vi "Microscopy.Circular Buffer (BRAM)_Array_Multi-Channel.vi"(0 "Input Write Data":T2=[0, 0, 0, 0], 1 "Acquisition Status In":T1, 2 "Read Data?":bool, 3 "Input Valid":bool, 5 "Acq Param Pre Trigger Samples":u16) -> (7 "Output Write Data":T2, 9 "Acquisition Status Out":T1, 10 "Output Valid":bool)   [LabVIEW 2014]
doc: "This VI maintains a circular buffer with user configurable buffer size.\nMaximum Buffer Size = 4096 (U32) elements\n\n<b> Delay = 1 Tick </b>"
uses:
  Adapter Module Specific/Multi-Channel Analog Input Data.ctl
  Acquisition Status.ctl
  <vilib>/Utility/error.llb/Clear Errors.vi
  <vilib>/rvi/Emulation/niFpgaSctlEmulationGetInTimedLoop.vi
  <vilib>/rvi/DataTransferAndStorage/Container/Common/niFpgaContainerGetUniqueNameForEmu.vi
  <vilib>/rvi/DataTransferAndStorage/Container/Common/niFpgaContainerSetEmuInfo.vi
  <vilib>/rvi/eio/common/nirviEmuReportErrorAndStop.vi
  <vilib>/rvi/Memory/Memory_Emulation/nirvimemoryEmulation.vi
  <vilib>/rvi/Memory/Memory_Emulation/nirvimemoryFastEmulation.vi
  <vilib>/rvi/Memory/Memory_Emulation/niFpgaMemoryEmulationCacheClearOnFirstRun.vi
  <vilib>/rvi/Memory/Memory_Emulation/nirvimemoryEmulationManagerCache_MakeExclusive.vi
  <vilib>/rvi/Memory/Memory_Emulation/niFpgaMemoryEmulationValidateCache.vi
  <vilib>/rvi/Memory/Memory_Emulation/nirvimemoryEmulationManagerCache_InsertValue.vi
  <vilib>/rvi/Memory/Memory_Emulation/nirvimemoryEmulationManagerCache_ReleaseExclusive.vi
  <vilib>/rvi/Memory/Memory_Emulation/nirvimemoryEmulationManagerCache_GetValue.vi
  <vilib>/rvi/Emulation/niFpgaEmulationIsFPGAContextNoSignature.vi
  <vilib>/rvi/Memory/Memory_Emulation/nirvimemoryEmulationManagerCache_SetValue.vi
  <vilib>/rvi/Emulation/niFpgaSctlEmulationResourceMgr.vi
  <vilib>/rvi/LocalResourceManager/LocalResourceManager.xnode
  <vilib>/rvi/DataTransferAndStorage/Container/XNode/niFpgaContainer.xnode
panel:
  # "Copyright 2014 Vidrio Technologies\nScanImage 5 software is licensed under the Apache License, Version 2.0 (the \"License\"); you may not use any files contained\nwithin the ScanImage 5 release except in compliance with the License. You may obtain a copy of the License at\n http://www.apache.org/licenses/LICENSE-2.0\nUnless required by applicable law or agreed to in writing, software distributed under the License is distributed on an\n\"AS IS\" BASIS, WITHOUT WARRANTIES OR CONDITIONS OF ANY KIND, either express or implied. See the License for the\n specific language governing permissions and limitations under the License."
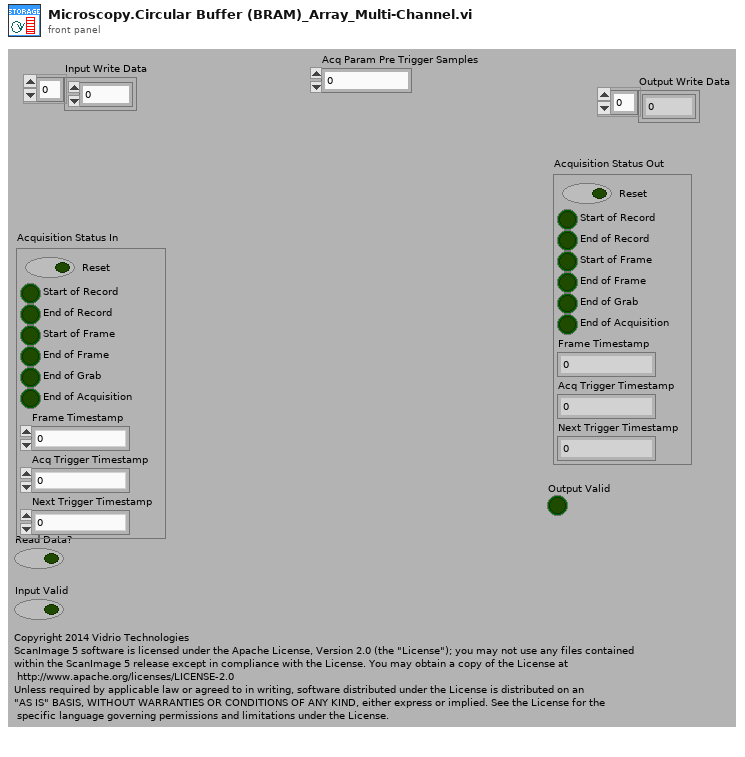
[diagram p1: front panel]
types:
  T1 = typedef "Acquisition Status.ctl" = cluster{"Reset":bool, "Start of Record":bool, "End of Record":bool, "Start of Frame":bool, "End of Frame":bool, "End of Grab":bool, "End of Acquisition":bool, "Frame Timestamp":u64, "Acq Trigger Timestamp":u64, "Next Trigger Timestamp":u64}
  T2 = typedef "Multi-Channel Analog Input Data.ctl" = i16[]
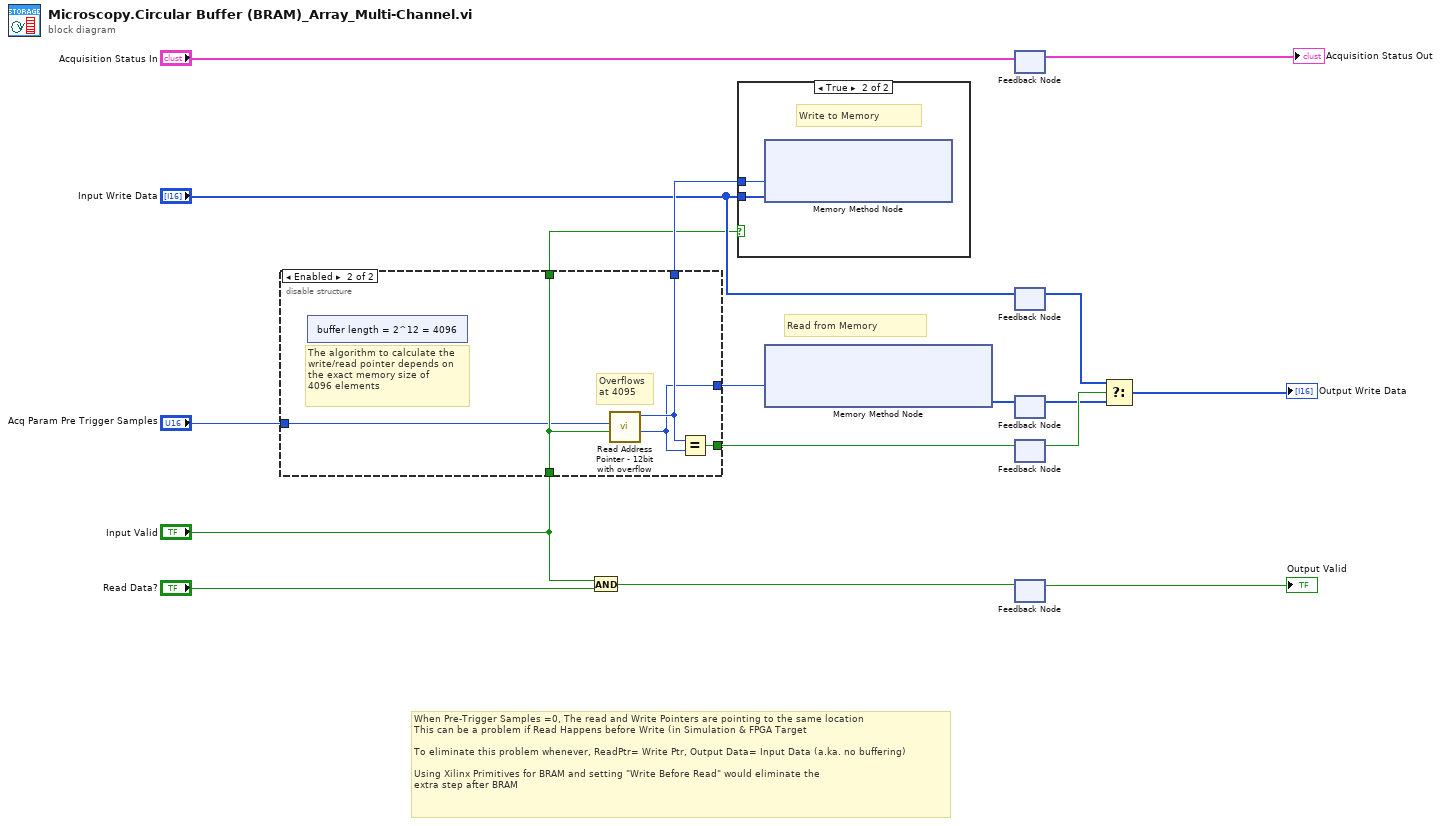
[diagram p0: block diagram]
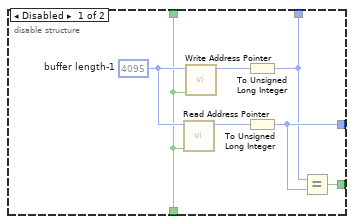
[diagram p2: hidden frame]
diagram:
  # "When Pre-Trigger Samples =0, The read and Write Pointers are pointing to the same location\nThis can be a problem if Read Happens before Write (in Simulation & FPGA Target\n\nTo eliminate this problem whenever, ReadPtr= Write Ptr, Output Data= Input Data (a.ka. no buffering)\n\nUsing Xilinx Primitives for BRAM and setting \"Write Before Read\" would eliminate the\nextra step after BRAM"
  # "Read from Memory"
  n1 = disable-structure shown="Enabled" {
    disable-tunnel: [w24 w26] -> w13
    disable-tunnel: [w23 w25] -> w11
    disable-tunnel: [w22 w27] -> w10
    disable-tunnel: "Input Valid" -> [w18 w29]
    disable-tunnel: [w18 w29] -> w2
    disable-tunnel: "Acq Param Pre Trigger Samples" -> [_ w28]
    frame Disabled {
      w19 = u16 4095  # buffer length-1
      n2 = call "Read Address Pointer.vi"("INC?"=w18, "rollover"=w19) -> ("count"=w21:u16)  [unwired: 9 in]
      n3 = call "Write Address Pointer.vi"("INC?"=w18, "rollover"=w19) -> ("count"=w20:u16)  [unwired: 9 in]
      n4 = To Unsigned Long Integer(number=w20) -> (unsigned 32bit integer=w22:u32)
      n5 = To Unsigned Long Integer(number=w21) -> (unsigned 32bit integer=w24:u32)
      n6 = Equal?(x=w22, y=w24) -> (x = y?=w23:bool)
    }
    frame Enabled {
      # "The algorithm to calculate the\nwrite/read pointer depends on\nthe exact memory size of\n4096 elements"
      # "Overflows\nat 4095"
      n7 = xnode "buffer length = 2^12 = 4096"() -> ()  [unwired: 1 out]
      n8 = call "Read Address Pointer - 12bit with overflow.vi"("INC?"=w29, "Read Pointer Offset"=w28) -> ("Read Pointer"=w26:u32, "Write Pointer"=w27:u32)  [unwired: 8 in]
      n9 = Equal?(x=w27, y=w26) -> (x = y?=w25:bool)
    }
  }
  n10 = And(x="Input Valid", y="Read Data?") -> (x .and. y?=w4:bool)
  n11 = case shown="True" w2 {
    tunnel: "Input Write Data" -> [_ w31]
    tunnel: w10 -> [_ w30]
    frame False {
    }
    frame True {
      # "Write to Memory"
      n12 = xnode ("Memory Method Node")("Address"=w30, "Data"=w31) -> ()  [unwired: 1 in, 1 out]
    }
  }
  n13 = xnode ("Memory Method Node")("Address"=w13) -> ("Data"=w17:i16[])  [unwired: 1 in, 1 out]
  n14 = feedback #1() -> (→"Acquisition Status Out":T1)  [unwired: 1 in]
  n15 = feedback-in #1("Acquisition Status In") -> ()
  n16 = feedback #2() -> (w9:T2)  [unwired: 1 in]
  n17 = feedback-in #2("Input Write Data") -> ()
  n18 = feedback #3() -> (w8:i16[])  [unwired: 1 in]
  n19 = feedback-in #3(w17) -> ()
  n20 = feedback #4() -> (w12:bool)  [unwired: 1 in]
  n21 = feedback-in #4(w11) -> ()
  n22 = feedback #5() -> (→"Output Valid":bool)  [unwired: 1 in]
  n23 = feedback-in #5(w4) -> ()
  n24 = Select(t=w9, s=w12, f=w8) -> (s? t:f=→"Output Write Data":T2)
